vi "Timer FGV with pause and resume.vi"(8 "Error In":errorcluster, 10 "Timeout / s":dbl, 11 "Command":T1) -> (0 "Error Out":errorcluster, 2 "Elapsed time / s":dbl, 3 "Finished?":bool)   [LabVIEW 2013]
doc: "This VI demonstrates how to build a timer with pause and resume functionality.\n\nThe VI is implemented as a non-blocking functional global variable (FGV).\n\nDr. Chris Empson\nSchool of Chemistry\nUniversity of Leeds\nUK\n\nc.j.empson@leeds.ac.uk\nTwitter: @monty_mcmont\nDownloaded from https://github.com/mcmont/LabVIEW_examples"
uses:
  Timer commands.ctl
panel:
  # "Timer with pause & resume.\n\nDr. Chris Empson\nSchool of Chemistry\nUniversity of Leeds\nUK\n\nc.j.empson@leeds.ac.uk\nTwitter: @monty_mcmont\nDownloaded from https://github.com/mcmont/LabVIEW_examples"
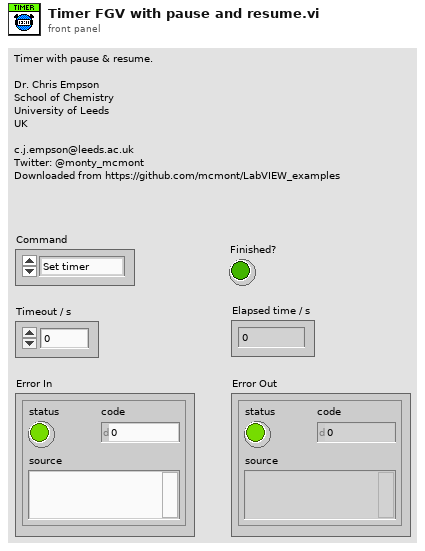
[diagram p1: front panel]
types:
  T1 = typedef "Timer commands.ctl" = enum16{"Set timer", "Check timer", "Pause timer", "Resume timer"}
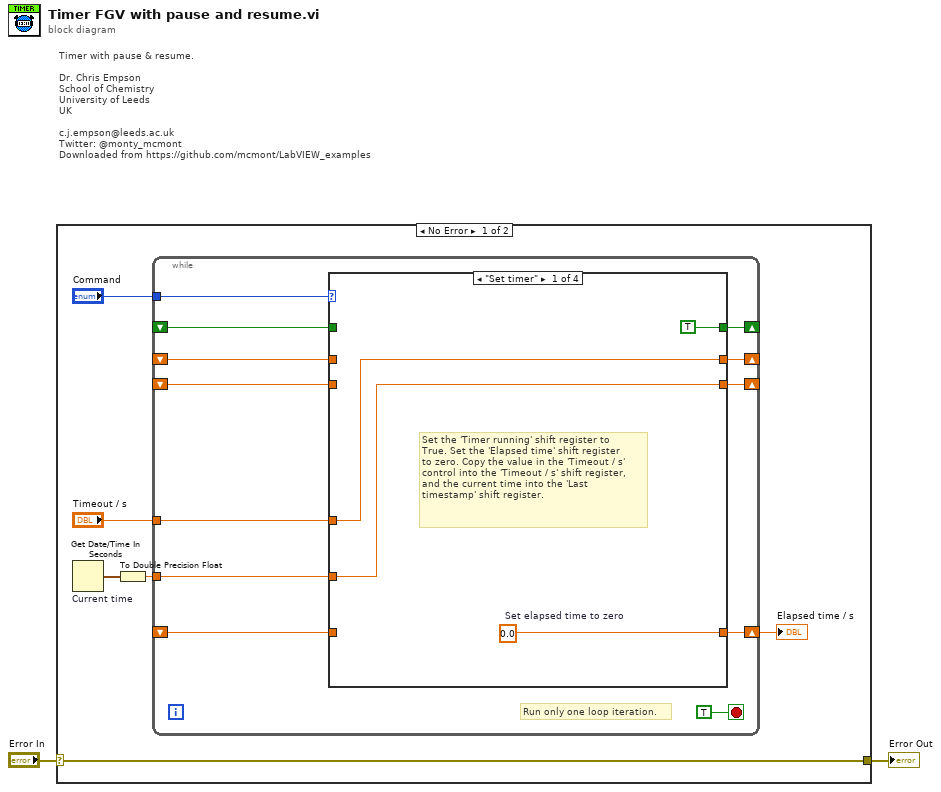
[diagram p0: block diagram]
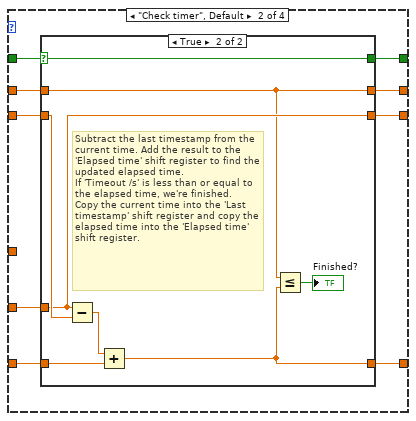
[diagram p2: hidden frame]
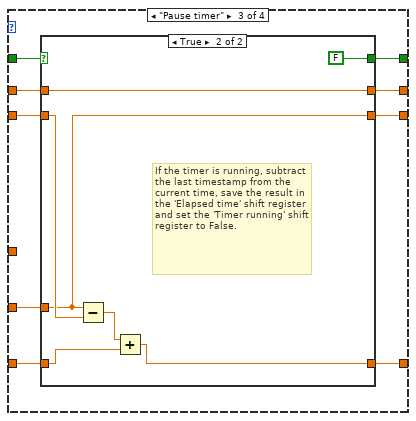
[diagram p4: hidden frame]
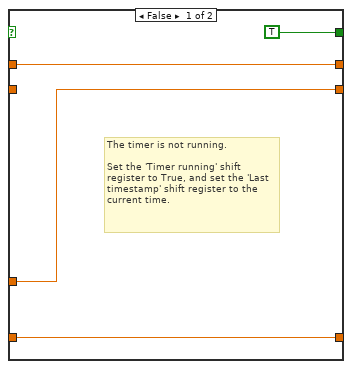
[diagram p7: hidden frame]
diagram:
  # "Timer with pause & resume.\n\nDr. Chris Empson\nSchool of Chemistry\nUniversity of Leeds\nUK\n\nc.j.empson@leeds.ac.uk\nTwitter: @monty_mcmont\nDownloaded from https://github.com/mcmont/LabVIEW_examples"
  n1 = case shown="No Error" "Error In" {
    selector: "Error In" -> [w8 w83]
    tunnel: [w8 w83] -> w1
    frame No Error {
      n2 = Get Date/Time In Seconds "Current time"() -> (seconds since 1Jan1904=w4:timestamp)
      n3 = To Double Precision Float(number=w4) -> (double precision float=w3:dbl)
      n4 = while {
        tunnel: "Command" -> [w19]
        tunnel: "Timeout / s" -> [w18]
        shift-right: [w16] -> _
        shift-left: _ -> [w17]
        shift-right: [w15] -> _
        shift-left: _ -> [w12]
        shift-right: [w14] -> _
        shift-left: _ -> [w11]
        shift-right: [w10] -> w5
        shift-left: _ -> [w13]
        tunnel: w3 -> [w9]
        stop <- TRUE stop-if-true
        # "Run only one loop iteration."
        n5 = case shown="\"Set timer\"" w19 {
          tunnel: w18 -> [w24 _ _ _]
          tunnel: w17 -> [_ w33 w50 w67]
          tunnel: [TRUE w32 w54 w74] -> w16
          tunnel: [w24 w30 w52 w72] -> w15
          tunnel: [w23 w28 w49 w70] -> w14
          tunnel: w13 -> [_ w27 w48 w69]
          tunnel: w12 -> [_ w31 w53 w73]
          tunnel: w11 -> [_ w29 w51 w71]
          tunnel: [w21 w26 w47 w68] -> w10
          tunnel: w9 -> [w23 w25 w46 w66]
          frame "Set timer" {
            w21 = 0.0  # Set elapsed time to zero
            # "Set the 'Timer running' shift register to \nTrue. Set the 'Elapsed time' shift register\nto zero. Copy the value in the 'Timeout / s'\ncontrol into the 'Timeout / s' shift register,\nand the current time into the 'Last\ntimestamp' shift register."
          }
          frame "Check timer", Default {
            n6 = case shown="True" w33 {
              selector: w33 -> [w37 w38]
              tunnel: [w37 w38] -> w32
              tunnel: w31 -> [w36 w40]
              tunnel: [w36 w40] -> w30
              tunnel: w29 -> [w35 w45]
              tunnel: [w35 w41] -> w28
              tunnel: w27 -> [w34 w43]
              tunnel: [w34 w39] -> w26
              tunnel: w25 -> [_ w41]
              frame False {
                # "The timer isn't running, so there's no\nneed to update the elapsed time."
              }
              frame True {
                # "Subtract the last timestamp from the current time. Add the result to the 'Elapsed time' shift register to find the updated elapsed time. \nIf 'Timeout /s' is less than or equal to the elapsed time, we're finished.\nCopy the current time into the 'Last timestamp' shift register and copy the elapsed time into the 'Elapsed time' shift register."
                n7 = Subtract(x=w41, y=w45) -> (x-y=w44:dbl)
                n8 = Add(x=w44, y=w43) -> (x+y=w39:dbl)
                n9 = Less Or Equal?(x=w40, y=w39) -> (x <= y?=→"Finished?":bool)
              }
            }
          }
          frame "Pause timer" {
            n10 = case shown="True" w50 {
              selector: w50 -> [w58 _]
              tunnel: [w58 FALSE] -> w54
              tunnel: w53 -> [w57 w64]
              tunnel: [w57 w64] -> w52
              tunnel: w51 -> [w56 w63]
              tunnel: [w56 w59] -> w49
              tunnel: w48 -> [w55 w61]
              tunnel: [w55 w60] -> w47
              tunnel: w46 -> [_ w59]
              frame False {
              }
              frame True {
                # "If the timer is running, subtract the last timestamp from the current time, save the result in the 'Elapsed time' shift register and set the 'Timer running' shift register to False."
                n11 = Subtract(x=w59, y=w63) -> (x-y=w62:dbl)
                n12 = Add(x=w62, y=w61) -> (x+y=w60:dbl)
              }
            }
          }
          frame "Resume timer" {
            n13 = case shown="True" w67 {
              selector: w67 -> [_ w79]
              tunnel: [TRUE w79] -> w74
              tunnel: w73 -> [w77 w82]
              tunnel: [w77 w82] -> w72
              tunnel: w71 -> [_ w81]
              tunnel: [w75 w81] -> w70
              tunnel: w69 -> [w76 w80]
              tunnel: [w76 w80] -> w68
              tunnel: w66 -> [w75 _]
              frame False {
                # "The timer is not running.\n\nSet the 'Timer running' shift register to True, and set the 'Last\ntimestamp' shift register to the\ncurrent time."
              }
              frame True {
                # "The timer is already running,\nso there's nothing to do."
              }
            }
          }
        }
      }
      "Elapsed time / s" <- w5
    }
    frame Error {
      # "An error condition was passed to this VI,\nso do nothing and pass on the error."
    }
  }
  "Error Out" <- w1
